vi "Set Strings from Ref.vi"(8 "error in (no error)":errorcluster, 9 "Language Index (0)":i32, 10 "GObj Refnum":refnum<vi>, 11 "WaveformGraph in":refnum<class "WaveformGraph.lvclass">) -> (0 "error out":errorcluster, 3 "WaveformGraph out":refnum<class "WaveformGraph.lvclass">)   [LabVIEW 2013, in "SET Project Data.lvlib" / "WaveformGraph.lvclass"]
uses:
  WaveformGraph.lvclass
  GraphChart/GraphChart.lvclass
  GObject/GObject.lvclass
  SET Project Data.lvlib
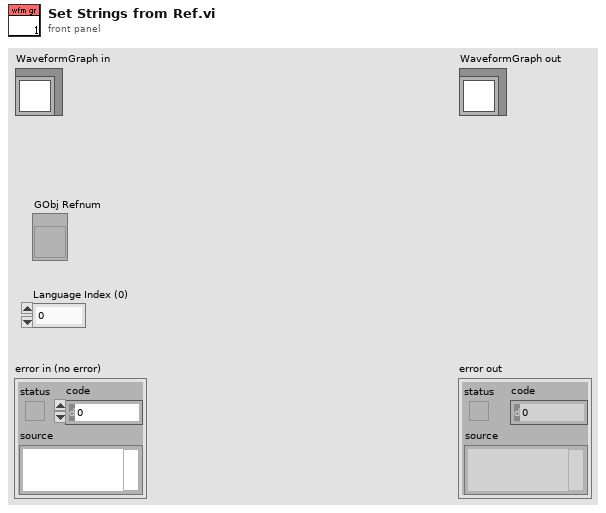
[diagram p1: front panel]
types:
  T1 = typedef "LVCursorListTypeDef.ctl" = cluster{"Name":string, "Color":u32, "Style":u8, "Point Style":u8, "Name Visible":bool, "Allow Drag":bool, "Cursor Mode":u32, "Plot":i32, "Index":i32, "Position":cluster{"X":dbl, "Y":dbl}, "X Scale":u32, "Y Scale":u32, "Watch Plots":i32[], "Watch All Plots":bool, "Plot Area":i32, "Label Offset":cluster{"X":dbl, "Y":dbl}}[]
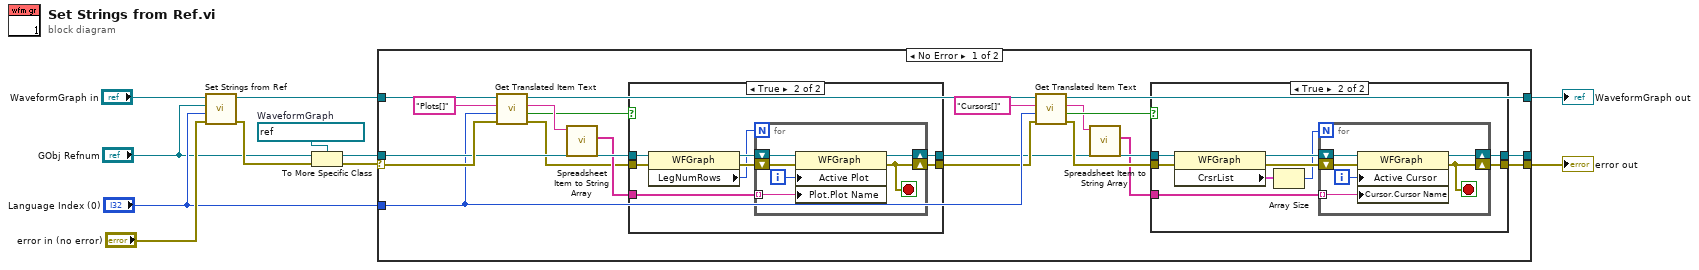
[diagram p0: block diagram]
diagram:
  w7 = refnum<vi> refnum  # WaveformGraph
  n1 = call-parent "Set Strings from Ref.vi"("error in (no error)"="error in (no error)", "Language Index (0)"="Language Index (0)", "GObj Refnum"="GObj Refnum", "GraphChart in"="WaveformGraph in") -> ("error out"=w5:errorcluster, "GraphChart out"=w6:refnum<class "WaveformGraph.lvclass">)  [unwired: 6 in]
  n2 = To More Specific Class(target class=w7, reference="GObj Refnum", error in=w5) -> (specific class reference=w9:refnum<vi>, error out=w8:errorcluster)
  n3 = case shown="No Error" w8 {
    selector: w8 -> [w28 w66]
    tunnel: w9 -> [w26 w65]
    tunnel: w6 -> [w30 w67]
    tunnel: "Language Index (0)" -> [w20 _]
    tunnel: [w16 w67] -> w2
    tunnel: [w13 w66] -> w1
    tunnel: [w12 w65] -> _
    frame No Error {
      n4 = call "Get Translated Item Text.vi"("error in (no error)"=w28, "LangIndex (0)"=w20, "ItemName"="Plots[]", "GObject in"=w30) -> ("error out"=w24:errorcluster, "Found?"=w27:bool, "Translated Text (ASCII)"=w29:string, "GObject out"=w22:refnum<class "WaveformGraph.lvclass">)  [unwired: 4 in]
      n5 = call "Spreadsheet Item to String Array.vi"("Spreadsheet Item (ASCII)"=w29) -> ("Strings [] (ASCII)"=w25:string[])  [unwired: 10 in]
      n6 = case shown="True" w27 {
        tunnel: w26 -> [w49 w55]
        tunnel: w25 -> [_ w58]
        tunnel: w24 -> [w50 w54]
        tunnel: [w50 w57] -> w19
        tunnel: [w49 w56] -> w17
        frame False {
        }
        frame True {
          n7 = property class="WFGraph"(reference=w55, error in=w54) -> (reference out=w53:refnum<vi>, error out=w52:errorcluster, "LegNumRows"=w51:u32)
          n8 = for {
            N: w51 -> [_]
            tunnel: w58 -> [w62] mode=indexing
            shift-right: [w61] -> w56
            shift-left: w53 -> [w64]
            shift-right: [w59] -> w57
            shift-left: w52 -> [w60]
            i -> [w63]
            stop <- w59 stop-if-true
            n9 = property class="WFGraph"(reference=w64, error in=w60, "Active Plot"=w63, "Plot.Plot Name"=w62) -> (reference out=w61:refnum<vi>, error out=w59:errorcluster)
          }
        }
      }
      n10 = call "Get Translated Item Text.vi"("error in (no error)"=w19, "LangIndex (0)"=w20, "ItemName"="Cursors[]", "GObject in"=w22) -> ("error out"=w18:errorcluster, "Found?"=w21:bool, "Translated Text (ASCII)"=w15:string, "GObject out"=w16:refnum<class "WaveformGraph.lvclass">)  [unwired: 4 in]
      n11 = call "Spreadsheet Item to String Array.vi"("Spreadsheet Item (ASCII)"=w15) -> ("Strings [] (ASCII)"=w14:string[])  [unwired: 10 in]
      n12 = case shown="True" w21 {
        tunnel: w17 -> [w32 w38]
        tunnel: w14 -> [_ w42]
        tunnel: w18 -> [w33 w37]
        tunnel: [w33 w41] -> w13
        tunnel: [w32 w40] -> w12
        frame False {
        }
        frame True {
          n13 = property class="WFGraph"(reference=w38, error in=w37) -> (reference out=w36:refnum<vi>, error out=w35:errorcluster, "CrsrList"=w39:T1)
          n14 = Array Size(array=w39) -> (size(s)=w34:i32)
          n15 = for {
            N: w34 -> [_]
            tunnel: w42 -> [w46] mode=indexing
            shift-right: [w45] -> w40
            shift-left: w36 -> [w48]
            shift-right: [w43] -> w41
            shift-left: w35 -> [w44]
            i -> [w47]
            stop <- w43 stop-if-true
            n16 = property class="WFGraph"(reference=w48, error in=w44, "Active Cursor"=w47, "Cursor.Cursor Name"=w46) -> (reference out=w45:refnum<vi>, error out=w43:errorcluster)
          }
        }
      }
    }
    frame Error {
    }
  }
  "error out" <- w1
  "WaveformGraph out" <- w2
